vi "Input-Output-DAQmx.vi"(7 "n samples\nper channel":i32=41200, 8 "Enable Output":bool, 9 "data":waveform(dbl)={"t0"=timestamp(0 s since 1904-01-01), "dt"=0.0, "Y"=[]}, 10 "task/channels in":refnum<k21>, 11 "Input Task In":refnum<k21>) -> (0 "error out":errorcluster, 1 "Input Data Sink":waveform(dbl), 2 "task out":refnum<k21>, 3 "Input task Out":refnum<k21>)   [LabVIEW 2022 SP3]
uses:
  <vilib>/Utility/error.llb/DialogType.ctl
  <vilib>/DAQmx/read.llb/DAQmx Read (Analog Wfm 1Chan NSamp).vi
  <vilib>/DAQmx/write.llb/DAQmx Write (Analog Wfm 1Chan NSamp).vi
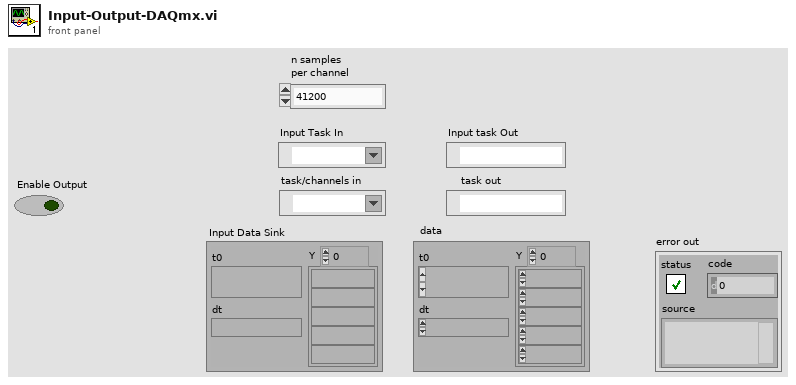
[diagram p1: front panel]
types:
  T1 = typedef "DialogType.ctl" = u16
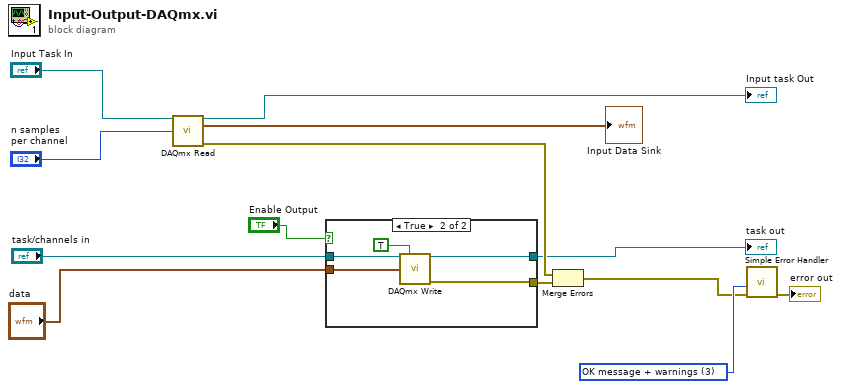
[diagram p0: block diagram]
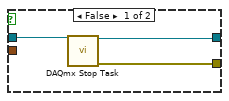
[diagram p2: hidden frame]
diagram:
  w11 = T1 3 items=["no dialog", "OK message", "continue or stop message", "OK message + warnings", "continue/stop + warnings"] ("type of dialog (OK msg:1)")
  n1 = call-poly <vilib>:"DAQmx Read.vi"("task/channels in"="Input Task In", "number of samples per channel"="n samples\nper channel") -> ("task out"=→"Input task Out":refnum<k21>, "data"=→"Input Data Sink":waveform(dbl), "error out"=w12:errorcluster)  [unwired: 11 in]
  n2 = case shown="True" "Enable Output" {
    tunnel: [w16 w21] -> w10
    tunnel: "task/channels in" -> [w15 w19]
    tunnel: [w14 w20] -> w4
    tunnel: "data" -> [_ w17]
    frame False {
      n3 = call <vilib>:"DAQmx Stop Task.vi"("task/channels in"=w15) -> ("task out"=w14:refnum<k21>, "error out"=w16:errorcluster)  [unwired: 13 in]
    }
    frame True {
      n4 = call-poly <vilib>:"DAQmx Write.vi"("task/channels in"=w19, "auto start"=TRUE, "data"=w17) -> ("task out"=w20:refnum<k21>, "error out"=w21:errorcluster)  [unwired: 10 in, 1 out]
    }
  }
  "task out" <- w4
  n5 = Merge Errors(w12, w10) -> (w9:errorcluster)
  n6 = call <vilib>:"Simple Error Handler.vi"("type of dialog (OK msg:1)"=w11, "error in (no error)"=w9) -> ("error out"=→"error out":errorcluster)  [unwired: 3 in, 4 out]
